vi "checktangent.vi"(6 "expect tangent":dbl, 7 "times":u16, 8 "down":dbl, 9 "up":dbl, 10 "sample sn":string[](array[string]), 11 "sample port":refnum<visa-resource-name>[](array[refnum])) -> (0 "tangnet":dbl[](array[numeric]), 1 "ok":bool, 2 "Array":bool[](array[boolean]))   [LabVIEW 2012]
uses:
  globalstatus.vi
panel:
  out "tangnet pool":dbl[][](array[numeric])
  out "count":u16
  in  "Enum":enum16{"excit", "get tangent"}(ring)
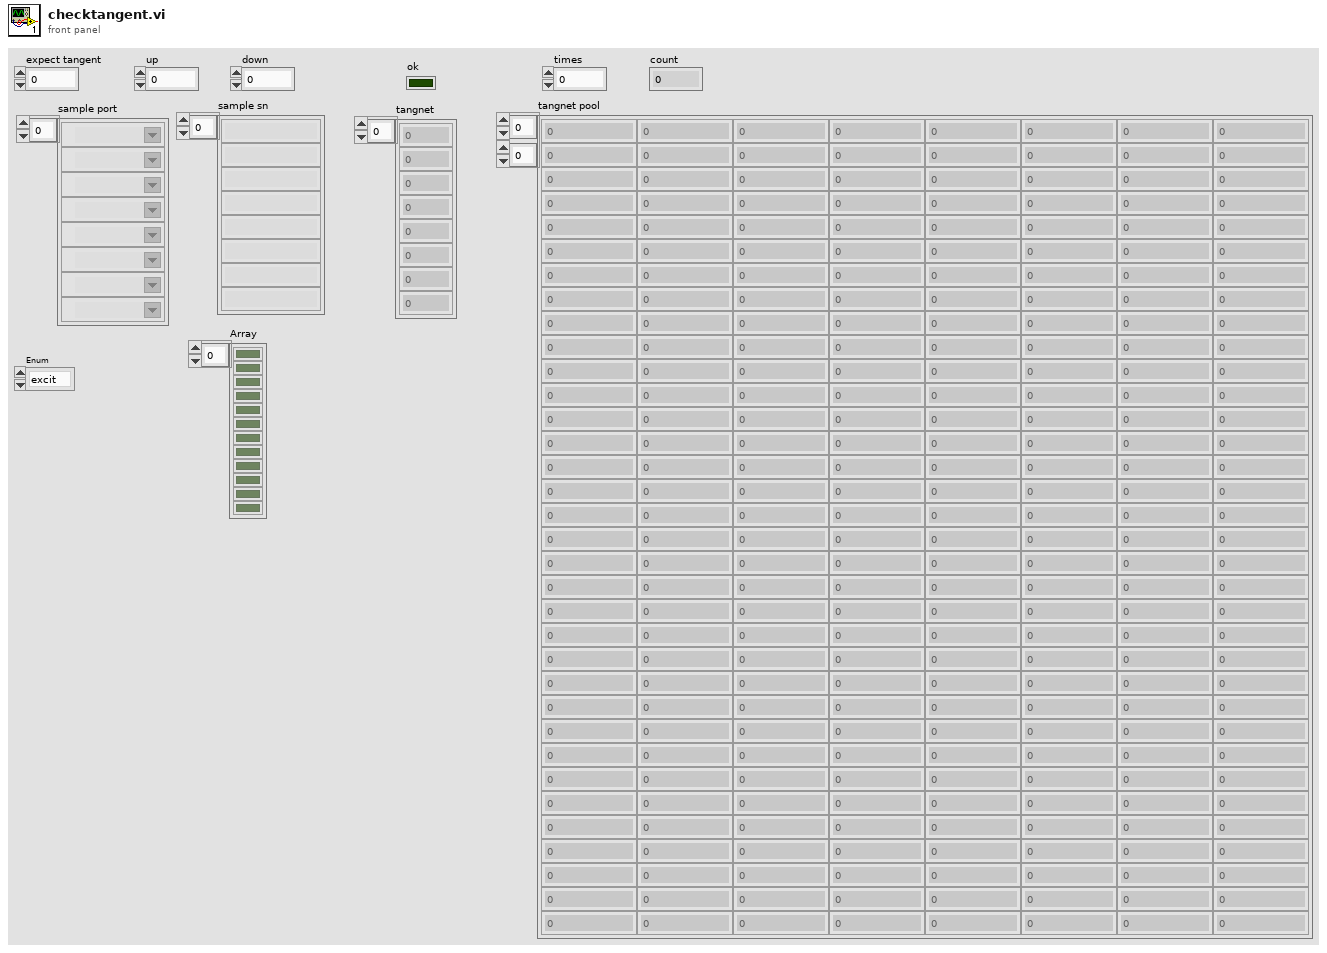
[diagram p1: front panel]
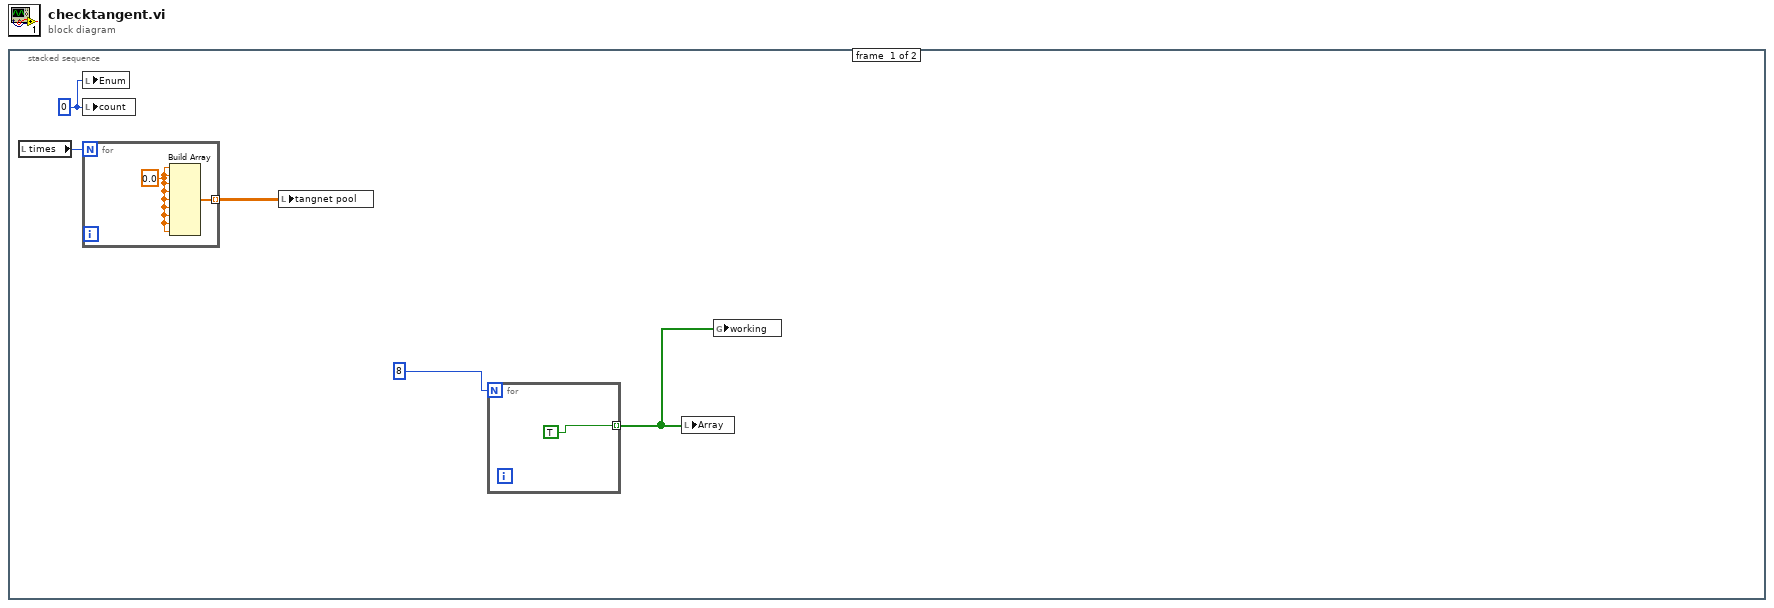
[diagram p0: block diagram]
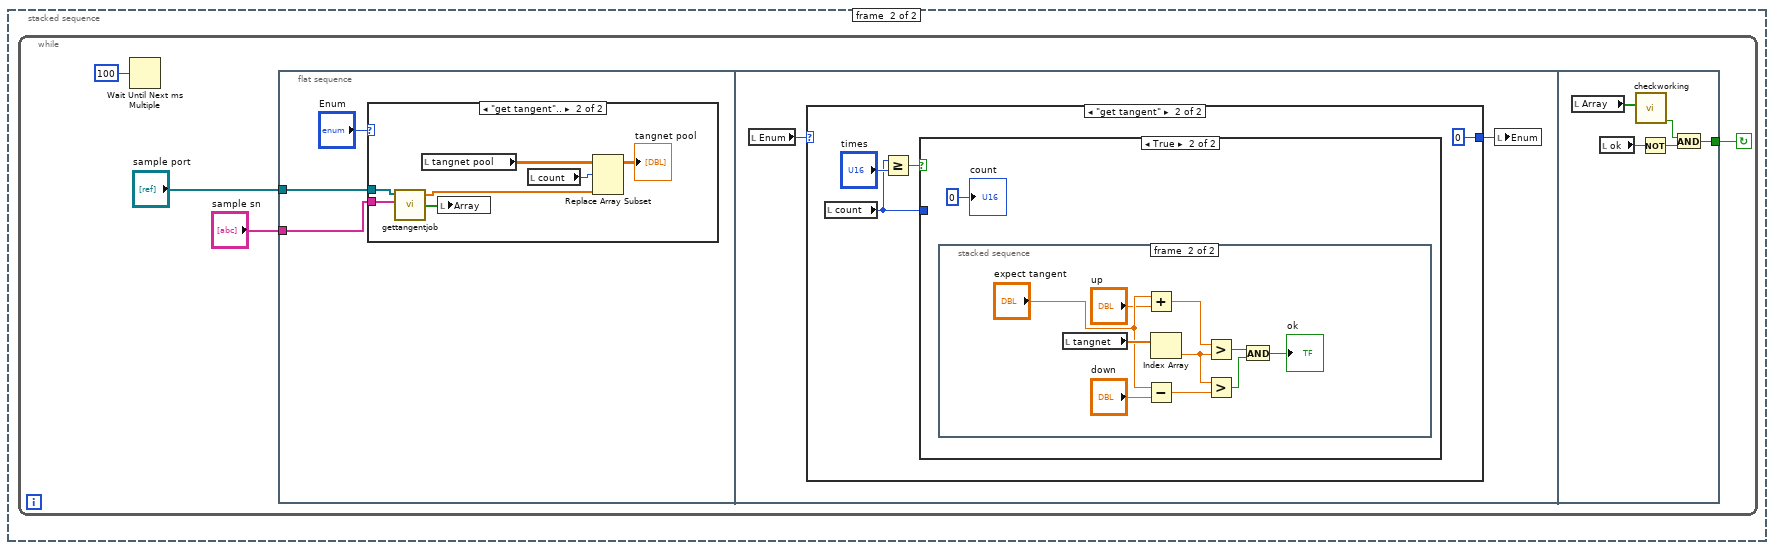
[diagram p2: hidden frame]
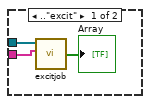
[diagram p3: hidden frame]
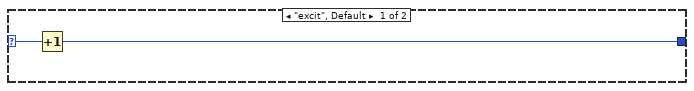
[diagram p4: hidden frame]
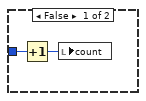
[diagram p5: hidden frame]
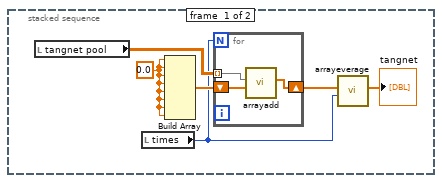
[diagram p6: hidden frame]
diagram:
  n1 = stacked-sequence {
    frame #0 {
      w3 = 0
      n2 = local read "times"() -> (w5:u16)
      n3 = local write "Enum"(w3) -> ()
      n4 = local write "count"(w3) -> ()
      n5 = for {
        N: w5 -> [_]
        tunnel: [w7] -> w4 mode=indexing
        w8 = 0.0
        n6 = Build Array(w8, w8, w8, w8, w8, w8, w8, w8, w8) -> (w7:dbl[])
      }
      n7 = local write "tangnet pool"(w4) -> ()
      n8 = for {
        N: 8 -> [_]
        tunnel: [TRUE] -> w1 mode=indexing
      }
      n9 = local write "Array"(w1) -> ()
      n10 = global write "globalstatus.vi" "working"(w1) -> ()
    }
    frame #1 {
      n11 = while {
        stop <- w9 continue-if-true
        n12 = Wait Until Next ms Multiple(millisecond multiple=100) -> ()  [unwired: 1 out]
        n13 = flat-sequence {
          tunnel: "sample port" -> [w15]
          tunnel: "sample sn" -> [w14]
          tunnel: [w58] -> w9
          frame #0 {
            n14 = case shown="\"get tangent\".." "Enum" {
              tunnel: w15 -> [w18 w25]
              tunnel: w14 -> [w17 w24]
              frame .."excit" {
                n15 = call "excitjob.vi"("sample port"=w18, "sample sn"=w17) -> ("Array"=→"Array":bool[])  [unwired: 5 in, 1 out]
              }
              frame "get tangent".. {
                n16 = call "gettangentjob.vi"("sample port"=w25, "sample sn"=w24) -> ("tangent"=w21:dbl[], "Array"=w23:bool[])  [unwired: 5 in]
                n17 = local read "tangnet pool"() -> (w22:dbl[][])
                n18 = local write "Array"(w23) -> ()
                n19 = local read "count"() -> (w20:u16)
                n20 = Replace Array Subset(array=w22, new element=w21, index (row)=w20) -> (→"tangnet pool":dbl[][])  [unwired: 1 in]
              }
            }
          }
          frame #1 {
            n21 = local read "Enum"() -> (w27:enum16{"excit", "get tangent"})
            n22 = case shown="\"get tangent\"" w27 {
              selector: w27 -> [w29 _]
              tunnel: [w28 0] -> w26
              frame "excit", Default {
                n23 = Increment(x=w29) -> (x+1=w28:enum16{"excit", "get tangent"})
              }
              frame "get tangent" {
                n24 = local read "count"() -> (w30:u16)
                n25 = Greater Or Equal?(x=w30, y="times") -> (x >= y?=w32:bool)
                n26 = case shown="True" w32 {
                  tunnel: w30 -> [w35 _]
                  frame False {
                    n27 = Increment(x=w35) -> (x+1=w34:u16)
                    n28 = local write "count"(w34) -> ()
                  }
                  frame True {
                    n29 = stacked-sequence {
                      frame #0 {
                        w40 = 0.0
                        n30 = local read "tangnet pool"() -> (w38:dbl[][])
                        n31 = local read "times"() -> (w37:u16)
                        n32 = Build Array(w40, w40, w40, w40, w40, w40, w40, w40) -> (w39:dbl[])
                        n33 = for {
                          N: w37 -> [_]
                          tunnel: w38 -> [w45] mode=indexing
                          shift-right: [w44] -> w42
                          shift-left: w39 -> [w43]
                          n34 = call "arrayadd.vi"("b"=w43, "a"=w45) -> ("c"=w44:dbl[])  [unwired: 9 in]
                        }
                        n35 = call "arrayeverage.vi"("divider"=w37, "in"=w42) -> ("out"=→"tangnet":dbl[])  [unwired: 9 in]
                      }
                      frame #1 {
                        n36 = local read "tangnet"() -> (w55:dbl[])
                        n37 = Add(x="expect tangent", y="up") -> (x+y=w51:dbl)
                        n38 = Subtract(x="expect tangent", y="down") -> (x-y=w50:dbl)
                        n39 = Index Array(array=w55) -> (element=w54:dbl)  [unwired: 1 in]
                        n40 = Greater?(x=w51, y=w54) -> (0:w47:bool)
                        n41 = Greater?(x=w54, y=w50) -> (0:w46:bool)
                        n42 = And(x=w47, y=w46) -> (x .and. y?=→"ok":bool)
                      }
                    }
                    "count" <- 0
                  }
                }
              }
            }
            n43 = local write "Enum"(w26) -> ()
          }
          frame #2 {
            n44 = local read "Array"() -> (w60:bool[])
            n45 = local read "ok"() -> (w57:bool)
            n46 = call "checkworking.vi"("Array"=w60) -> ("Boolean"=w59:bool)  [unwired: 8 in]
            n47 = Not(x=w57) -> (.not. x?=w56:bool)
            n48 = And(x=w59, y=w56) -> (x .and. y?=w58:bool)
          }
        }
      }
    }
  }
